vi "CRYExponent Apply to Units.vi"(10 "Exponent to apply":dbl=1.0 format="%.2f", 11 "Unit in":string) -> (3 "Unit out":string)   [LabVIEW 2013]
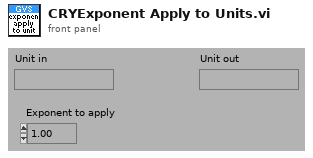
[diagram p1: front panel]
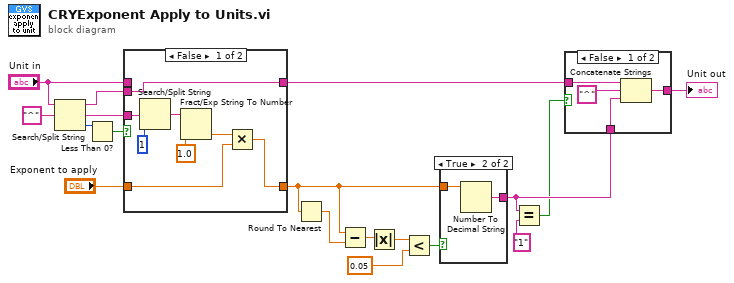
[diagram p0: block diagram]
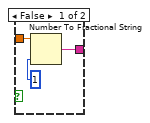
[diagram p3: hidden frame]
diagram:
  n1 = Search/Split String(string="Unit in", search string/char (-)="^") -> (substring before match=w12:string, match + rest of string=w13:string, offset of match=w17:i32)  [unwired: 1 out]
  n2 = Less Than 0?(x=w17) -> (x < 0?=w16:bool)
  n3 = case shown="False" w16 {
    tunnel: "Exponent to apply" -> [w21 w27]
    tunnel: "Unit in" -> [_ w28]
    tunnel: w13 -> [w26 _]
    tunnel: w12 -> [w20 _]
    tunnel: [w20 w28] -> w6
    tunnel: [w19 w27] -> w5
    frame False {
      n4 = Search/Split String(string=w26, offset (0)=1) -> (match + rest of string=w24:string)  [unwired: 3 out]
      n5 = Fract/Exp String To Number(string=w24, default (0 dbl)=1.0) -> (number=w22:dbl)  [unwired: 3 out]
      n6 = Multiply(x=w22, y=w21) -> (x*y=w19:dbl)
    }
    frame True {
    }
  }
  n7 = Round To Nearest(number=w5) -> (nearest integer value=w7:dbl)
  n8 = Subtract(x=w5, y=w7) -> (x-y=w8:dbl)
  n9 = Absolute Value(x=w8) -> (abs(x)=w9:dbl)
  n10 = Less?(x=w9, y=0.05) -> (x < y?=w11:bool)
  n11 = case shown="True" w11 {
    tunnel: w5 -> [w31 w33]
    tunnel: [w29 w32] -> w3
    frame False {
      n12 = Number To Fractional String(number=w31, precision (6)=i16 1) -> (F-format string=w29:string)  [unwired: 2 out]
    }
    frame True {
      n13 = Number To Decimal String(number=w33) -> (decimal integer string=w32:string)  [unwired: 1 out]
    }
  }
  n14 = Equal?(x=w3, y="1") -> (x = y?=w1:bool)
  n15 = case shown="False" w1 {
    tunnel: w6 -> [w37 w38]
    tunnel: [w36 w38] -> w4
    tunnel: w3 -> [w35 _]
    frame False {
      n16 = Concatenate Strings(w37, "^", w35) -> (w36:string)
    }
    frame True {
    }
  }
  "Unit out" <- w4
